vi "read_file1.vi"(4 "error in":errorcluster, 7 "file":path) -> (0 "error out":errorcluster, 1 "lowercase file ext":string, 2 "Elements":string[](array[string]), 3 "File Path":path)   [LabVIEW 2010]
uses:
  <vilib>/Utility/xml.llb/Read From XML File(array).vi
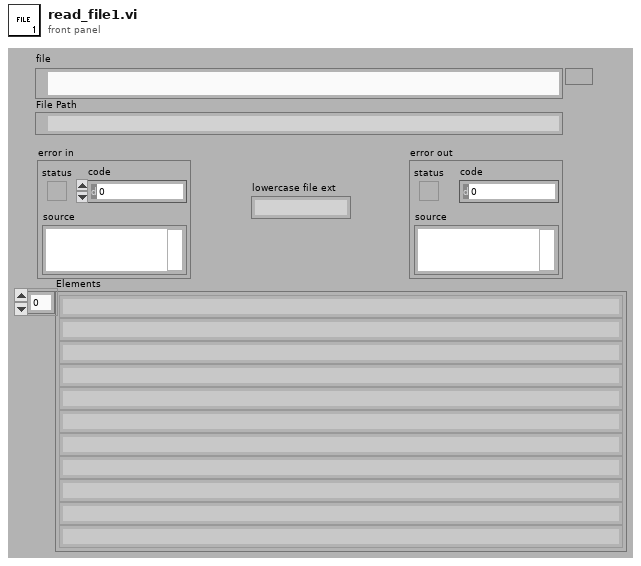
[diagram p1: front panel]
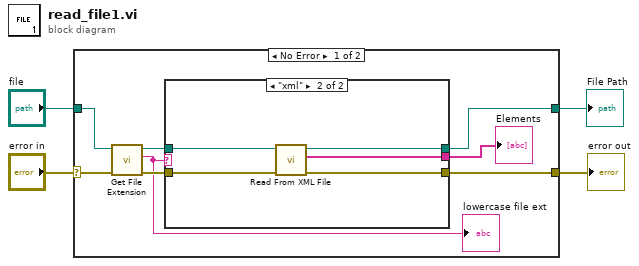
[diagram p0: block diagram]
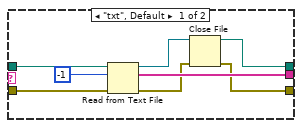
[diagram p2: hidden frame]
diagram:
  n1 = case shown="No Error" "error in" {
    selector: "error in" -> [w5 w27]
    tunnel: "file" -> [w9 w26]
    tunnel: [w8 w26] -> w3
    tunnel: [w6 w27] -> w2
    frame No Error {
      n2 = call <vilib>:"Get File Extension.vi"("error in (no error)"=w5, "file"=w9) -> ("error out"=w12:errorcluster, "lowercase file extension"=w10:string, "dup file"=w11:path)  [unwired: 6 in, 1 out]
      "lowercase file ext" <- w10
      n3 = case shown="\"xml\"" w10 {
        tunnel: [w18 w25] -> w7
        tunnel: w11 -> [w20 w24]
        tunnel: w12 -> [w19 w23]
        tunnel: [w14 w22] -> w8
        tunnel: [w13 w21] -> w6
        frame "txt", Default {
          n4 = Read from Text File(file (use dialog)=w20, count=-1, error in=w19) -> (refnum out=w15:refnum<file>, text=w18:string[], error out=w16:errorcluster)  [unwired: 1 in, 1 out]
          n5 = Close File(refnum=w15, error in=w16) -> (path=w14:path, error out=w13:errorcluster)
        }
        frame "xml" {
          n6 = call-poly <vilib>:"Read From XML File.vi"("error in (no error)"=w23, "XML File Path"=w24) -> ("error out"=w21:errorcluster, "XML Elements"=w25:string[], "XML File Path(duplicate)"=w22:path)  [unwired: 7 in]
        }
      }
      "Elements" <- w7
    }
    frame Error {
    }
  }
  "File Path" <- w3
  "error out" <- w2
